vi "HiPOT.vi"(6 "Setting":T1={"dc voltage"=100, "high limit"=4e-07, "test time(s)"=3.0, "Channel"=""} {"high limit" format="%#_10f"}, 8 "error in":errorcluster, 9 "HiPOT Ref":string, 10 "HiPOT ClassName":string="Hioki BT4560B.lvclass", 11 "Base Path":path=path "C:/GitHub/OOP_OPC UA/Sequence/CodeModules/HAL/Concrete") -> (0 "error out":errorcluster={"status"=TRUE, "code"=-1073807346, "source"="VISA Open in APS-7000 Series.lvlib:Initialize.vi->Concrete.lvlib:APS7050.lvclass:Initialise.vi->Check objects.vi"}, 3 "Measurements":dbl)   [LabVIEW 2021]
uses:
  HAL/Harware Abstraction/HiPOT/HiPOT.lvclass
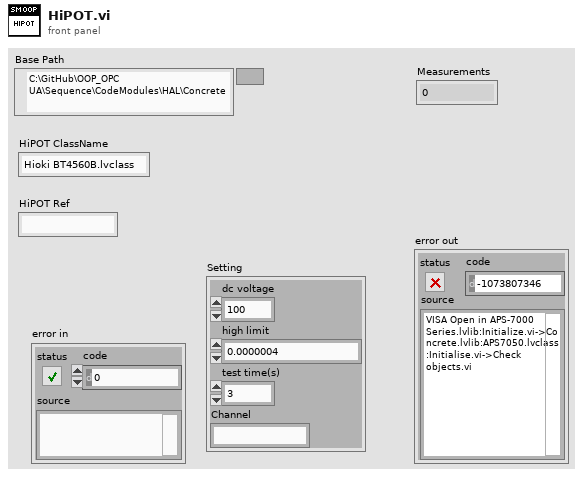
[diagram p1: front panel]
types:
  T1 = cluster{"dc voltage":i32, "high limit":dbl, "test time(s)":dbl, "Channel":string}
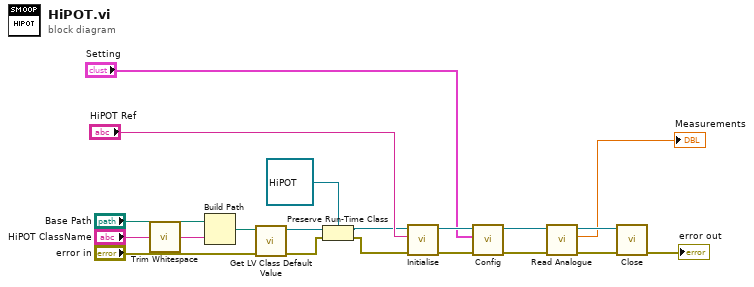
[diagram p0: block diagram]
diagram:
  n1 = call <vilib>:"Trim Whitespace.vi"("string"="HiPOT ClassName") -> ("trimmed string"=w18:string)  [unwired: 1 in]
  n2 = Build Path(base path="Base Path", name or relative path=w18) -> (appended path=w16:path)
  n3 = call <vilib>:"Get LV Class Default Value.vi"("error in (no error)"="error in", "class path"=w16) -> ("error out"=w15:errorcluster, "object"=w19:refnum<class>)  [unwired: 8 in]
  n4 = Preserve Run-Time Class(object in=w19, error in=w15, 2:refnum<class "HiPOT.lvclass"> refnum ("HAL.lvlib:HiPOT.lvclass")) -> (object out=w13:refnum<class "HiPOT.lvclass">, error out=w12:errorcluster)
  n5 = call-dynamic "Initialise.vi"("error in (no error)"=w12, "Instrument Ref"="HiPOT Ref", "Instrument in"=w13) -> ("error out"=w8:errorcluster, "Instrument out"=w7:refnum<class "HiPOT.lvclass">)  [unwired: 7 in]
  n6 = call-dynamic "Config.vi"("error in (no error)"=w8, "Setting"="Setting", "HiPOT in"=w7) -> ("error out"=w5:errorcluster, "HiPOT out"=w4:refnum<class "HiPOT.lvclass">)  [unwired: 7 in]
  n7 = call-dynamic "Read Analogue.vi"("error in (no error)"=w5, "PS in"=w4) -> ("error out"=w3:errorcluster, "Measurements"=→"Measurements":dbl, "PS out"=w2:refnum<class "HiPOT.lvclass">)  [unwired: 7 in]
  n8 = call-dynamic "Close.vi"("error in (no error)"=w3, "Instrument in"=w2) -> ("error out"=→"error out":errorcluster)  [unwired: 8 in, 1 out]
